vi "Actor Core.vi"(8 "error in":errorcluster, 11 "Grayscale in":refnum<class "Grayscale.lvclass">) -> (0 "error out":errorcluster, 3 "Actor out":refnum<class "Actor.lvclass">)   [LabVIEW 2016, in "Tests.lvlib" / "Grayscale.lvclass"]
doc: "This VI converts RGB Image to Grayscale Image."
uses:
  Grayscale.lvclass
  C:/Program Files (x86)/National Instruments/LabVIEW 2016/vi.lib/ActorFramework/Actor/Actor.lvclass
  <vilib>/ActorFramework/Actor/Actor.lvclass
  Grayscale Messages/New Image Msg/New Image Grayscale Msg.lvclass
  C:/Users/Achu/Desktop/2015/Image Acquisition/Image Acquisition Messages/Image Msg/Image Msg.lvclass
  Controls/Grayscale States.ctl
  Grayscale.lvclass/Grayscale.ctl
  <vilib>/vision/Image Controls.llb/IMAQ Image.ctl
  <vilib>/ActorFramework/Actor/Actor.lvclass/Actor.ctl
  <vilib>/ActorFramework/Message Enqueuer/Message Enqueuer.lvclass/Message Enqueuer.ctl
  Controller/Controller Messages/Request Image Msg/Request Image Msg.lvclass/Request Image Msg.ctl
  <vilib>/ActorFramework/Report Error Msg/Report Error Msg.lvclass/Report Error Msg.ctl
  <vilib>/ActorFramework/Message Enqueuer/Init from Existing Queue.vi
  <vilib>/ActorFramework/Message Enqueuer/Enqueue.vi
  Controller/Controller Messages/Request Image Msg/Request Image Msg.lvclass
  C:/Program Files (x86)/National Instruments/LabVIEW 2016/vi.lib/ActorFramework/Message/Message.lvclass
  <vilib>/ActorFramework/Report Error Msg/Report Error Msg.lvclass
  Grayscale Messages/Stop Grayscale Actor Msg/Stop Grayscale Actor Msg.lvclass
  <vilib>/ActorFramework/Stop Msg/Stop Msg.lvclass
  <vilib>/ActorFramework/Message Priority Queue/Priority Enqueue.vi
  Tests.lvclass
  <vilib>/ActorFramework/Message Enqueuer/Message Enqueuer.lvclass
  <vilib>/vision/NI_Vision_Development_Module.lvlib
panel:
  in  "Help Button":bool
  in  "Apply Grayscale":bool
  in  "Tests.lvlib:New Image Msg.lvclass":refnum<class "New Image Grayscale Msg.lvclass">
  in  "Send Image Request":bool
  out "Image":T1(plugin-control)
  # "Grayscale Image Viewer"
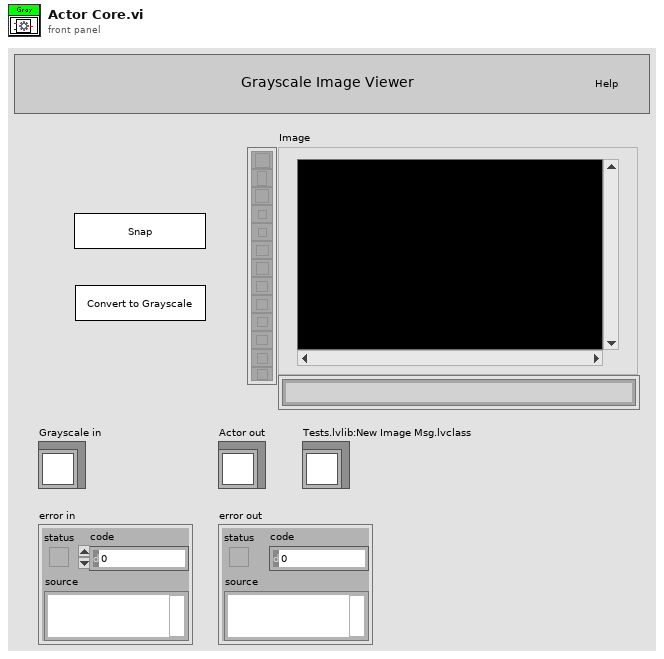
[diagram p1: front panel]
types:
  T1 = typedef "IMAQ Image.ctl" = refnum<image>
  T2 = typedef "Grayscale States.ctl" = enum16{"Poll UI", "Initialize", "Send Image Request", "Image", "Apply Grayscale", "Error", "Exit"}
  T3 = enum8{"Enabled", "Disabled", "Disabled and Grayed Out"}
  T4 = typedef "Image Type" = u32
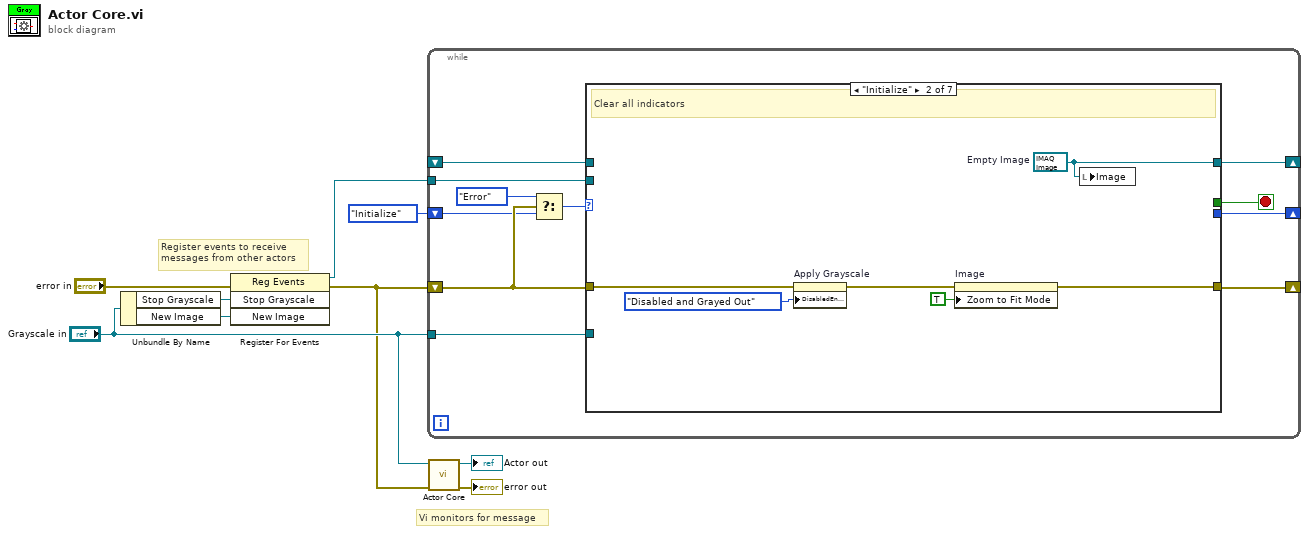
[diagram p0: block diagram]
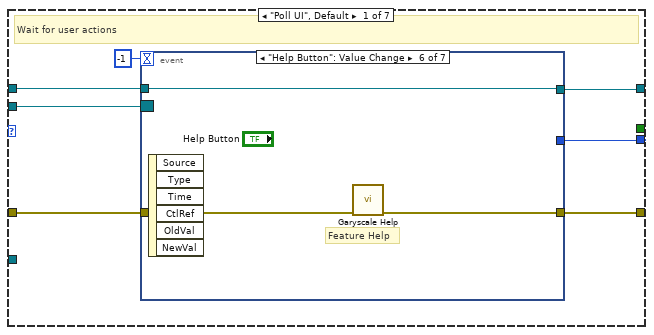
[diagram p2: hidden frame]
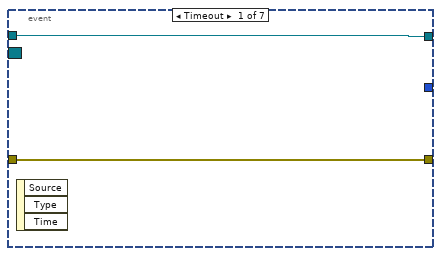
[diagram p3: hidden frame]
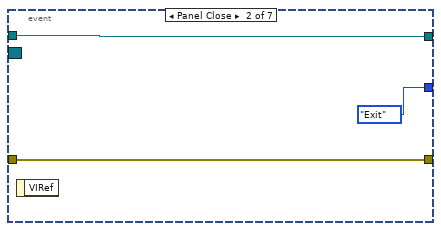
[diagram p4: hidden frame]
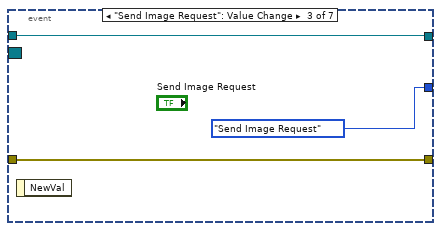
[diagram p5: hidden frame]
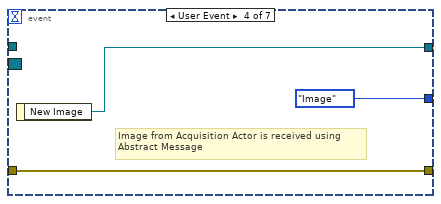
[diagram p6: hidden frame]
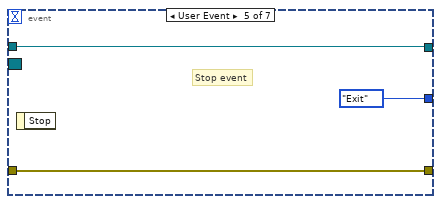
[diagram p7: hidden frame]
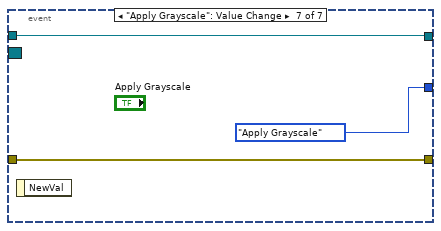
[diagram p8: hidden frame]
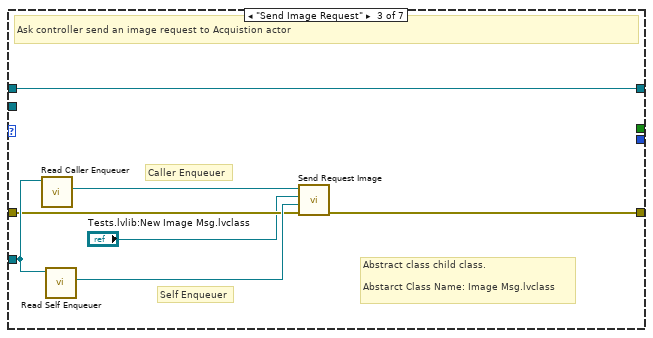
[diagram p9: hidden frame]
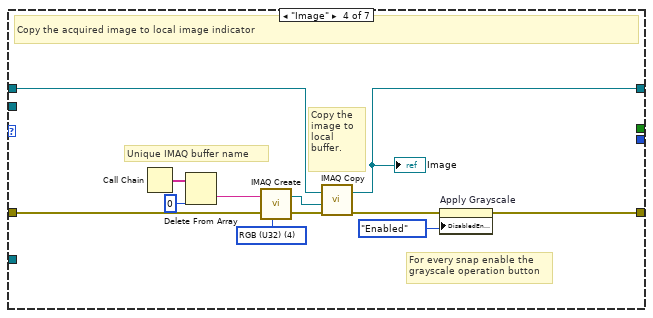
[diagram p10: hidden frame]
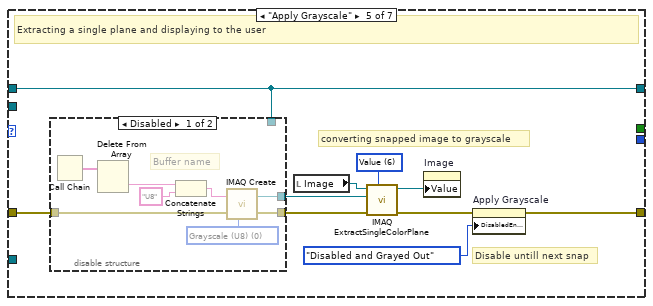
[diagram p11: hidden frame]
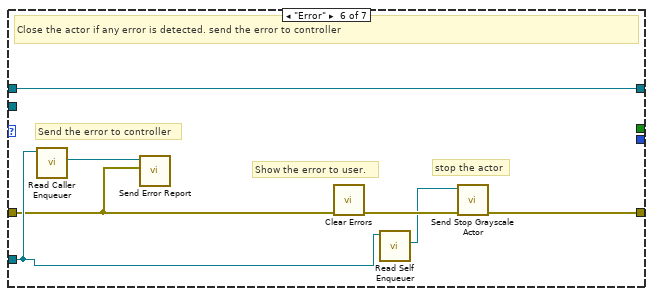
[diagram p13: hidden frame]
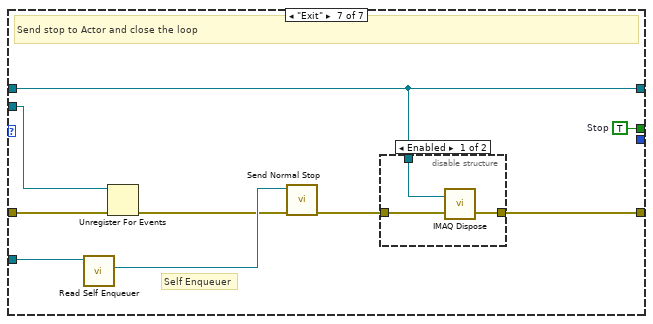
[diagram p14: hidden frame]
diagram:
  # "Vi monitors for message"
  # "Register events to receive\nmessages from other actors"
  n1 = Unbundle By Name("Grayscale in") -> ("Stop Grayscale"=w8:refnum<user-event>, "New Image"=w4:refnum<user-event>)
  n2 = register-events(error in="error in", w8, w4) -> (reference out=w7:refnum<event-registration>, error out=w1:errorcluster)  [unwired: 1 in]
  n3 = while {
    tunnel: w7 -> [w20]
    tunnel: "Grayscale in" -> [w19]
    shift-right: [w15] -> _
    shift-left: Grayscale_States."Initialize" -> [w11]
    shift-right: [w17] -> _
    shift-left: _ -> [w16]
    shift-right: [w18] -> _
    shift-left: w1 -> [w13]
    stop <- w14 stop-if-true
    n4 = Select(t=Grayscale_States."Error", s=w13, f=w11) -> (s? t:f=w10:T2)
    n5 = case shown="\"Initialize\"" w10 {
      tunnel: w20 -> [w27 _ _ _ _ _ w103]
      tunnel: w19 -> [_ _ w57 _ _ w95 w108]
      tunnel: w13 -> [w23 w52 w56 w69 w82 w93 w105]
      tunnel: [w22 w48 w55 w66 w77 w96 w101] -> w18
      tunnel: [w26 w53 w60 w62 w73 w99 w100] -> w17
      tunnel: w16 -> [w25 _ w60 w63 w73 w99 w100]
      tunnel: [w24 _ _ _ _ _ _] -> w15
      tunnel: [_ _ _ _ _ _ w106] -> w14
      frame "Poll UI", Default {
        # "Wait for user actions"
        n6 = event shown="[5] \"Help Button\": Value Change" {
          selector: w27 -> [_ _ _ _ _ _ _]
          dyn-events: _ -> [_ _ _ _ _ _ _]
          timeout: -1 -> [_ _ _ _ _ _ _]
          tunnel: [w29 w32 w35 w38 w41 w44 w47] -> w26
          tunnel: w25 -> [w29 w32 w35 _ w41 w44 w47]
          tunnel: [_ Grayscale_States."Exit" Grayscale_States."Send Image Request" Grayscale_States."Image" Grayscale_States."Exit" _ Grayscale_States."Apply Grayscale"] -> w24
          tunnel: w23 -> [w28 w30 w33 w36 w40 w43 w45]
          tunnel: [w28 w30 w33 w36 w40 w42 w45] -> w22
          event Timeout {
            n7 = event-data() -> ()  [unwired: 1 in, 3 out]
          }
          event Panel Close {
            n8 = event-data() -> ()  [unwired: 1 in, 1 out]
          }
          event "Send Image Request": Value Change {
            n9 = event-data() -> ()  [unwired: 1 in, 1 out]
          }
          event User Event {
            # "Image from Acquisition Actor is received using\nAbstract Message"
            n10 = event-data() -> ("New Image"=w38:T1)  [unwired: 1 in]
          }
          event User Event {
            # "Stop event"
            n11 = event-data() -> ()  [unwired: 1 in, 1 out]
          }
          event "Help Button": Value Change {
            # "Feature Help"
            n12 = event-data() -> ()  [unwired: 1 in, 6 out]
            n13 = call "Garyscale Help.vi"("error in (no error)"=w43) -> ("error out"=w42:errorcluster)  [unwired: 10 in]
          }
          event "Apply Grayscale": Value Change {
            n14 = event-data() -> ()  [unwired: 1 in, 1 out]
          }
        }
      }
      frame "Initialize" {
        w53 = T1 refnum  # Empty Image
        # "Clear all indicators"
        n15 = property on="Apply Grayscale" class="Bool"(error in=w52, "DisabledEnum"=T3."Disabled and Grayed Out" ("Disabled")) -> (error out=w49:errorcluster)  [unwired: 1 in, 1 out]
        n16 = property on="Image" class="ImageControl"(error in=w49, "Zoom to Fit Mode"=TRUE) -> (error out=w48:errorcluster)  [unwired: 1 in, 1 out]
        n17 = local write "Image"(w53) -> ()
      }
      frame "Send Image Request" {
        # "Self Enqueuer"
        # "Caller Enqueuer"
        # "Abstract class child class.\n\nAbstarct Class Name: Image Msg.lvclass"
        # "Ask controller send an image request to Acquistion actor"
        n18 = call <vilib>:"Read Caller Enqueuer.vi"("Actor"=w57) -> ("Caller Enqueuer"=w58:refnum<class "Message Enqueuer.lvclass">)  [unwired: 10 in]
        n19 = call <vilib>:"Read Self Enqueuer.vi"("Actor"=w57) -> ("Self Enqueuer"=w59:refnum<class "Message Enqueuer.lvclass">)  [unwired: 10 in]
        n20 = call "Send Request Image.vi"("error in (no error)"=w56, "Enqueuer"=w59, "Image Acquisition.lvlib:Image Msg.lvclass"="Tests.lvlib:New Image Msg.lvclass", "Message Enqueuer"=w58) -> ("error out"=w55:errorcluster)  [unwired: 6 in, 1 out]
      }
      frame "Image" {
        w68 = T4 4 items=["Grayscale (U8)", "Grayscale (I16)", "Grayscale (SGL)", "Complex (CSG)", "RGB (U32)", "HSL (U32)", "RGB (U64)", "Grayscale (U16)"] ("Image Type")
        # "Copy the image to\nlocal\nbuffer."
        # "For every snap enable the \ngrayscale operation button"
        # "Unique IMAQ buffer name"
        # "Copy the acquired image to local image indicator"
        n21 = Call Chain() -> (call chain=w71:string[])
        n22 = Delete From Array(array=w71, index=0) -> (deleted portion=w70:string)  [unwired: 1 in, 1 out]
        n23 = call "IMAQ Create"("Image Name"=w70, "Image Type"=w68, "error in (no error)"=w69) -> ("New Image"=w72:T1, "error out"=w65:errorcluster)  [unwired: 2 in]
        n24 = call "IMAQ Copy"("error in (no error)"=w65, "Image Dst"=w72, "Image Src"=w63) -> ("error out"=w64:errorcluster, "Image Dst Out"=w62:T1)  [unwired: 3 in]
        "Image" <- w62
        n25 = property on="Apply Grayscale" class="Bool"(error in=w64, "DisabledEnum"=T3."Enabled" ("Disabled")) -> (error out=w66:errorcluster)  [unwired: 1 in, 1 out]
      }
      frame "Apply Grayscale" {
        w81 = 6 items=["Red", "Green", "Blue", "Hue", "Saturation", "Luminance", "Value", "Intensity"] ("Color Plane")
        # "Disable untill next snap"
        # "converting snapped image to grayscale"
        # "Extracting a single plane and displaying to the user"
        n26 = disable-structure shown="Disabled" {
          disable-tunnel: w82 -> [w88 w91]
          disable-tunnel: [w84 w91] -> w80
          disable-tunnel: [w83 w92] -> w79
          disable-tunnel: w73 -> [_ w92]
          frame Disabled {
            w87 = T4 0 items=["Grayscale (U8)", "Grayscale (I16)", "Grayscale (SGL)", "Complex (CSG)", "RGB (U32)", "HSL (U32)", "RGB (U64)", "Grayscale (U16)"] ("Image Type")
            # "Buffer name"
            n27 = Call Chain() -> (call chain=w90:string[])
            n28 = Delete From Array(array=w90) -> (deleted portion=w89:string)  [unwired: 2 in, 1 out]
            n29 = Concatenate Strings(w89, "U8" ("string")) -> (w86:string)
            n30 = call "IMAQ Create"("Image Name"=w86, "Image Type"=w87, "error in (no error)"=w88) -> ("New Image"=w83:T1, "error out"=w84:errorcluster)  [unwired: 2 in]
          }
          frame Enabled {
          }
        }
        n31 = local read "Image"() -> (w75:T1)
        n32 = call "IMAQ ExtractSingleColorPlane"("Color Plane"=w81, "error in (no error)"=w80, "Image Dst"=w79, "Image Src"=w75) -> ("error out"=w78:errorcluster, "Image Dst Out"=w74:T1)  [unwired: 6 in]
        n33 = property on="Image" class="ImageControl"("Value"=w74) -> ()  [unwired: 2 in, 2 out]
        n34 = property on="Apply Grayscale" class="Bool"(error in=w78, "DisabledEnum"=T3."Disabled and Grayed Out" ("Disabled")) -> (error out=w77:errorcluster)  [unwired: 1 in, 1 out]
      }
      frame "Error" {
        # "stop the actor"
        # "Send the error to controller"
        # "Show the error to user."
        # "Close the actor if any error is detected. send the error to controller"
        n35 = call <vilib>:"Read Caller Enqueuer.vi"("Actor"=w95) -> ("Caller Enqueuer"=w98:refnum<class "Message Enqueuer.lvclass">)  [unwired: 10 in]
        n36 = call <vilib>:"Send Error Report.vi"("Error From Sender"=w93, "Message Enqueuer"=w98) -> ()  [unwired: 9 in, 1 out]
        n37 = call <vilib>:"Clear Errors.vi"("error in (no error)"=w93) -> ("error out"=w97:errorcluster)  [unwired: 5 in, 1 out]
        n38 = call <vilib>:"Read Self Enqueuer.vi"("Actor"=w95) -> ("Self Enqueuer"=w94:refnum<class "Message Enqueuer.lvclass">)  [unwired: 10 in]
        n39 = call "Send Stop Grayscale Actor.vi"("error in (no error)"=w97, "Message Enqueuer"=w94) -> ("error out"=w96:errorcluster)  [unwired: 8 in, 1 out]
      }
      frame "Exit" {
        w106 = TRUE  # Stop
        # "Self Enqueuer"
        # "Send stop to Actor and close the loop"
        n40 = call <vilib>:"Read Self Enqueuer.vi"("Actor"=w108) -> ("Self Enqueuer"=w107:refnum<class "Message Enqueuer.lvclass">)  [unwired: 10 in]
        n41 = Unregister For Events(event registration refnum=w103, error in=w105) -> (error out=w104:errorcluster)
        n42 = call <vilib>:"Send Normal Stop.vi"("error in (no error)"=w104, "Message Enqueuer"=w107) -> ("error out"=w102:errorcluster)  [unwired: 9 in]
        n43 = disable-structure shown="Enabled" {
          disable-tunnel: w102 -> [w111 w112]
          disable-tunnel: [w110 w112] -> w101
          disable-tunnel: w100 -> [w109 _]
          frame Enabled {
            n44 = call "IMAQ Dispose"("Image"=w109, "error in (no error)"=w111) -> ("error out"=w110:errorcluster)  [unwired: 4 in]
          }
          frame Disabled {
          }
        }
      }
    }
  }
  n45 = call-parent "Actor Core.vi"("error in"=w1, "Actor in"="Grayscale in") -> ("error out"=→"error out":errorcluster, "Actor out"=→"Actor out":refnum<class "Actor.lvclass">)  [unwired: 8 in]
